vi "管理员面板.vi"() -> ()   [LabVIEW 2019]
panel:
  out "错误输出 3":errorcluster caption="错误输出"
  out "Row":i32
  out "Column":i32
  out "error out 7":errorcluster
  out "当前选择的用户为":string
  in  "重置密码":bool
  in  "删除用户":bool
  out "成员名单":string[][](table)
  out "成员名单1":string[][](array[string])
  out "error out 4":errorcluster
  in  "返回":bool
  # "欢迎来到管理员面板"
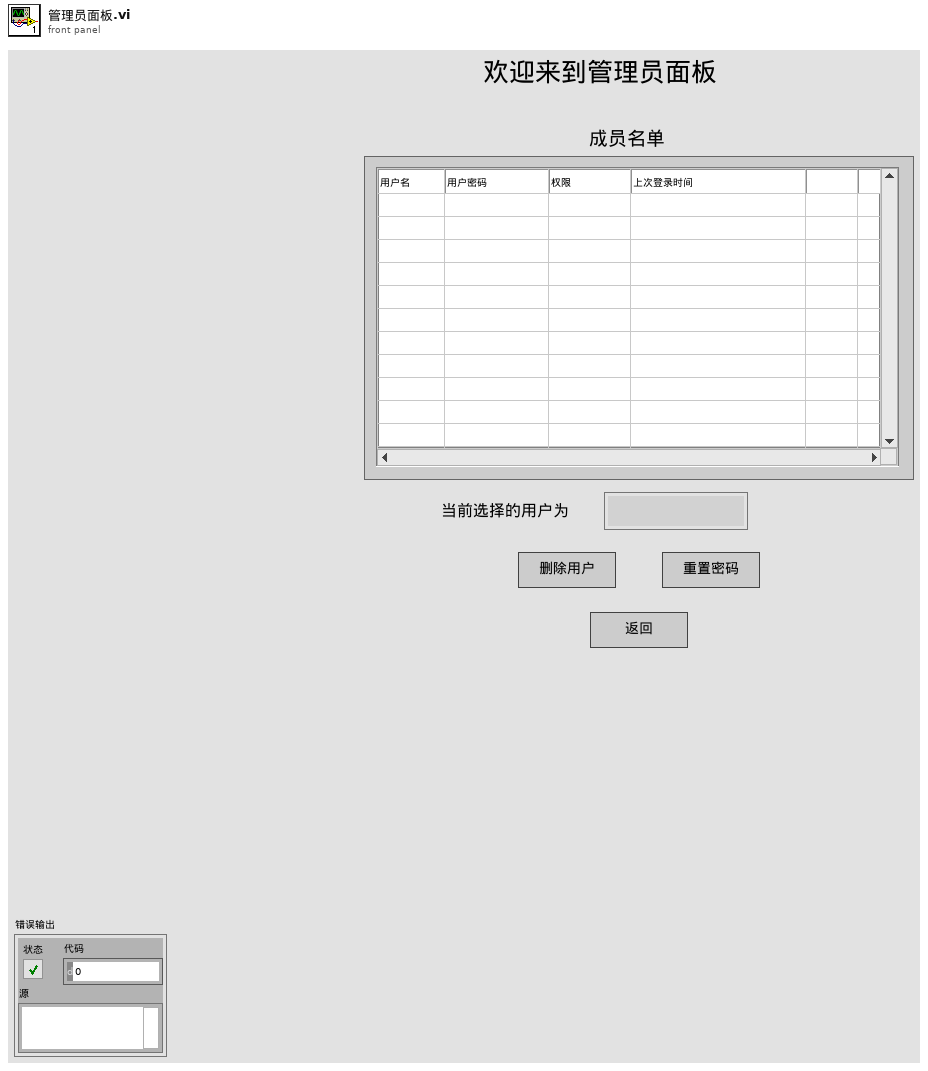
[diagram p1: front panel]
types:
  T1 = cluster{"Read Access":enum8{"Allowed", "Required", "None"}, "Write Access":enum8{"Allowed", "Required", "None"}}
  T2 = typedef "LVPoint32TypeDef.ctl" = cluster{"Horizontal":i32, "Vertical":i32}
  T3 = typedef "LVRowAndColumnTypeDef.ctl" = cluster{"Row":i32, "Column":i32}
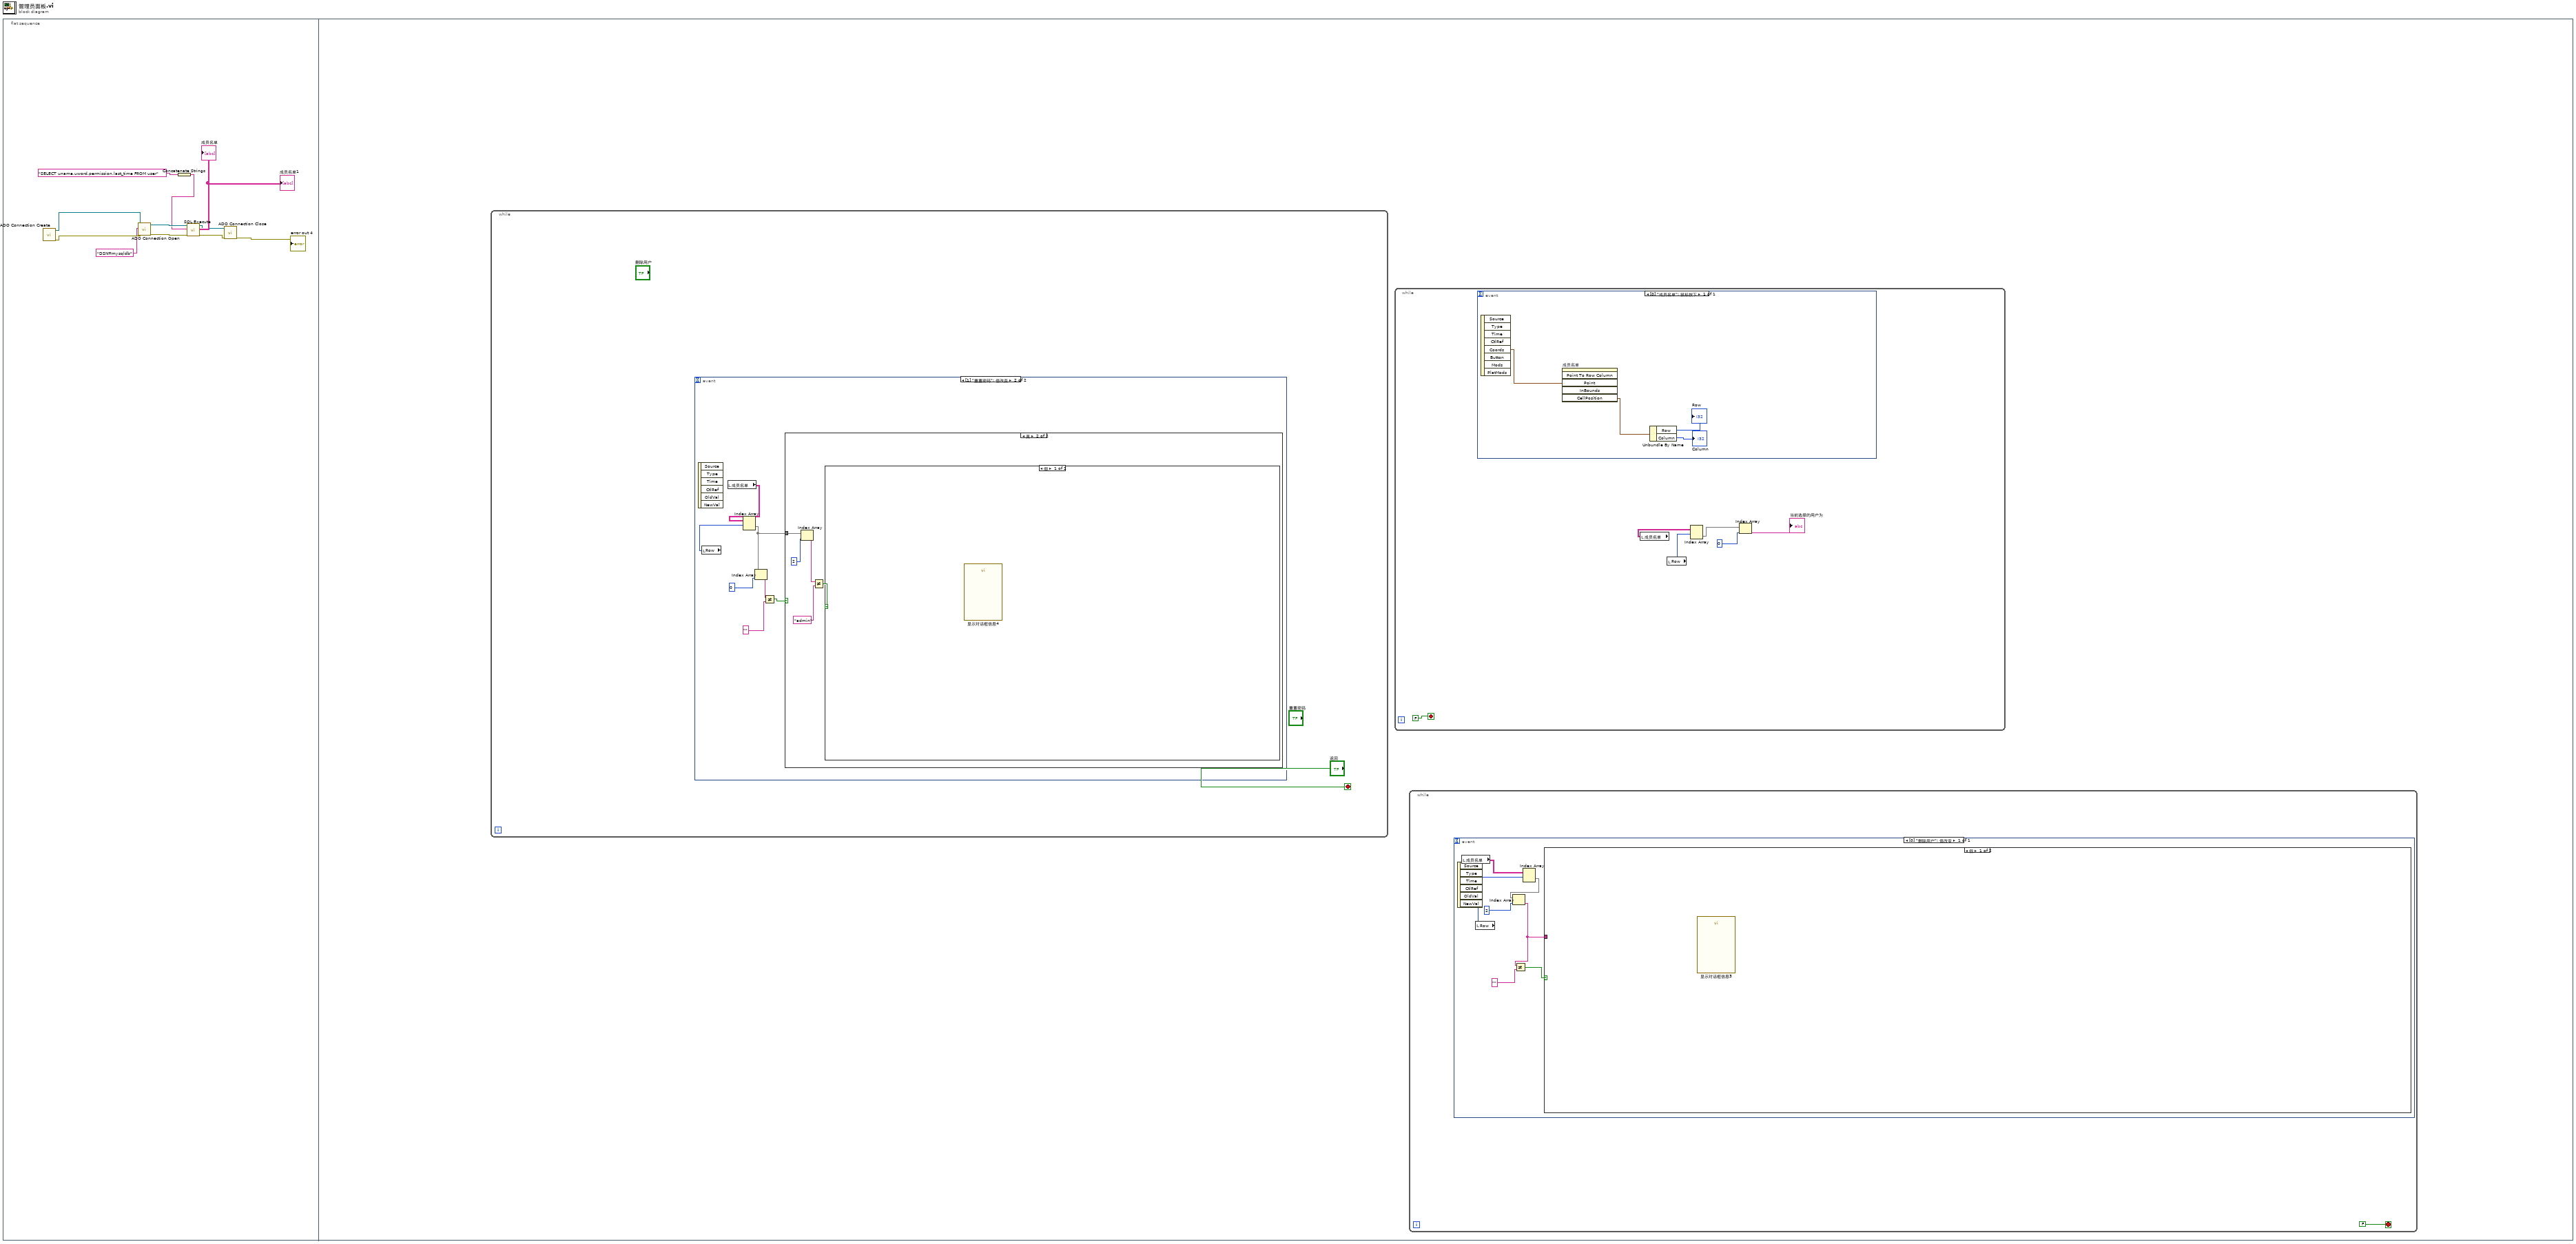
[diagram p0: block diagram]
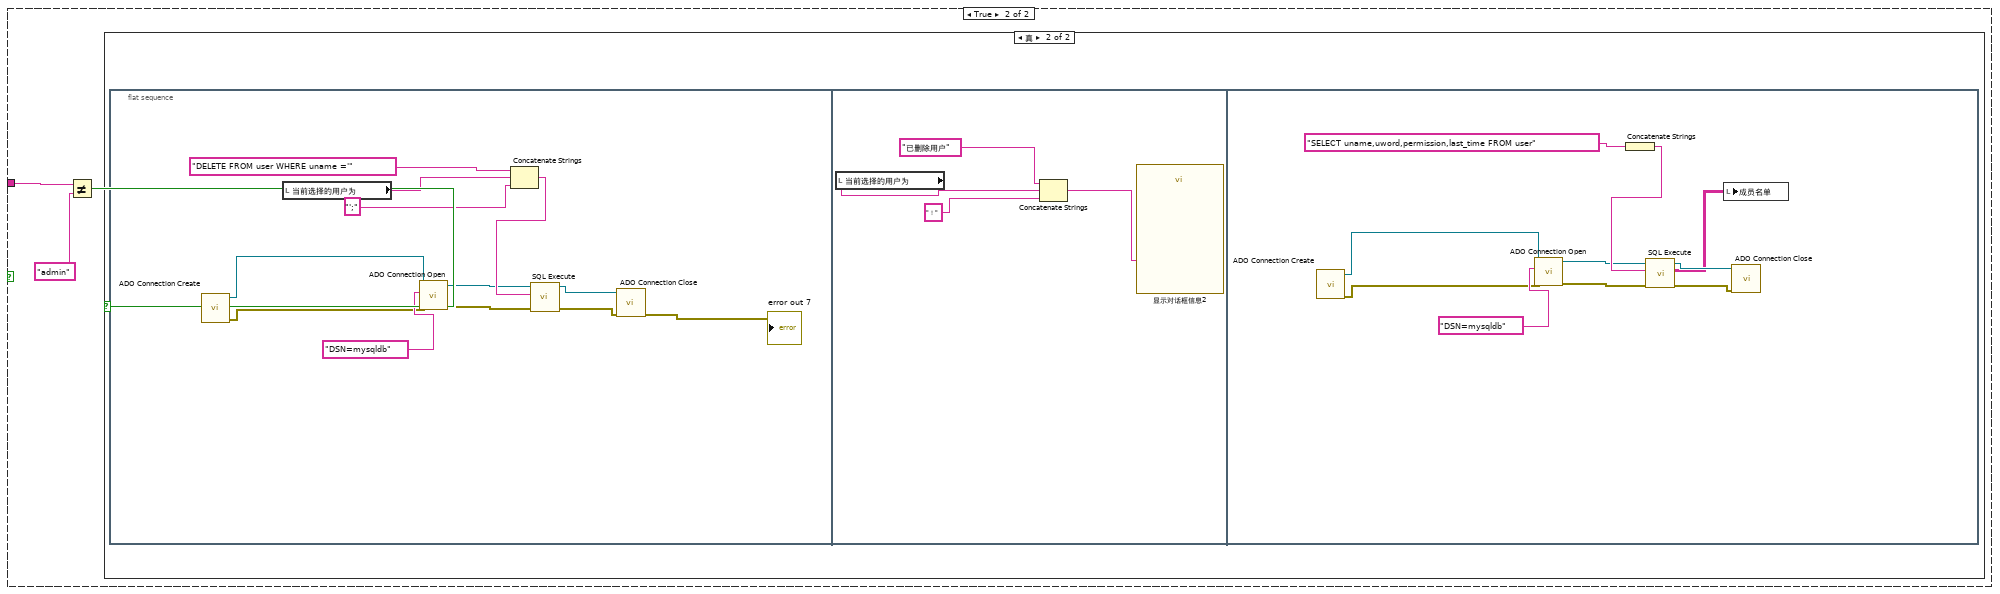
[diagram p2: hidden frame]
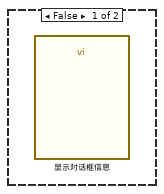
[diagram p3: hidden frame]
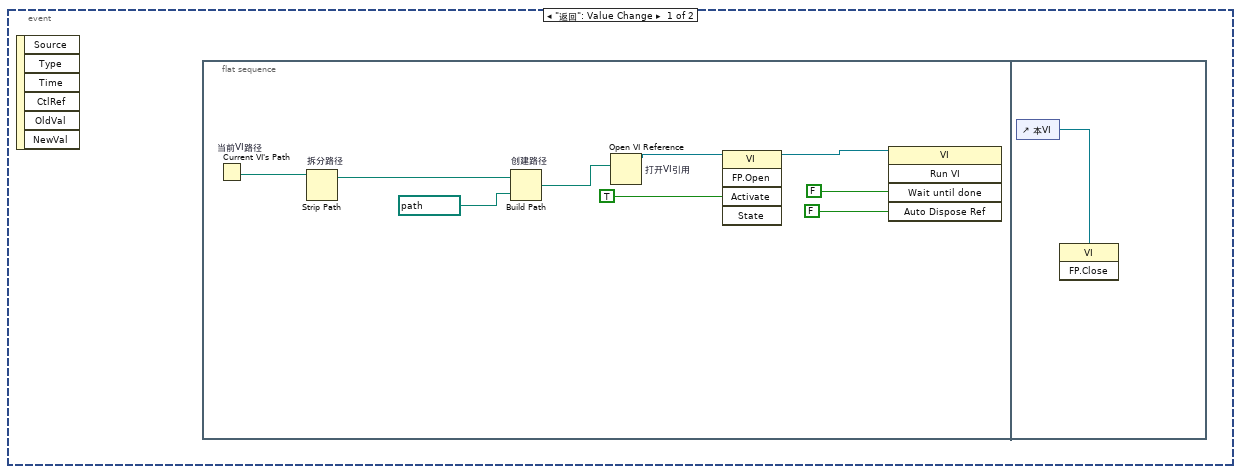
[diagram p4: hidden frame]
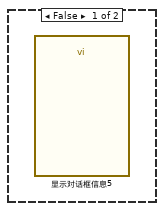
[diagram p5: hidden frame]
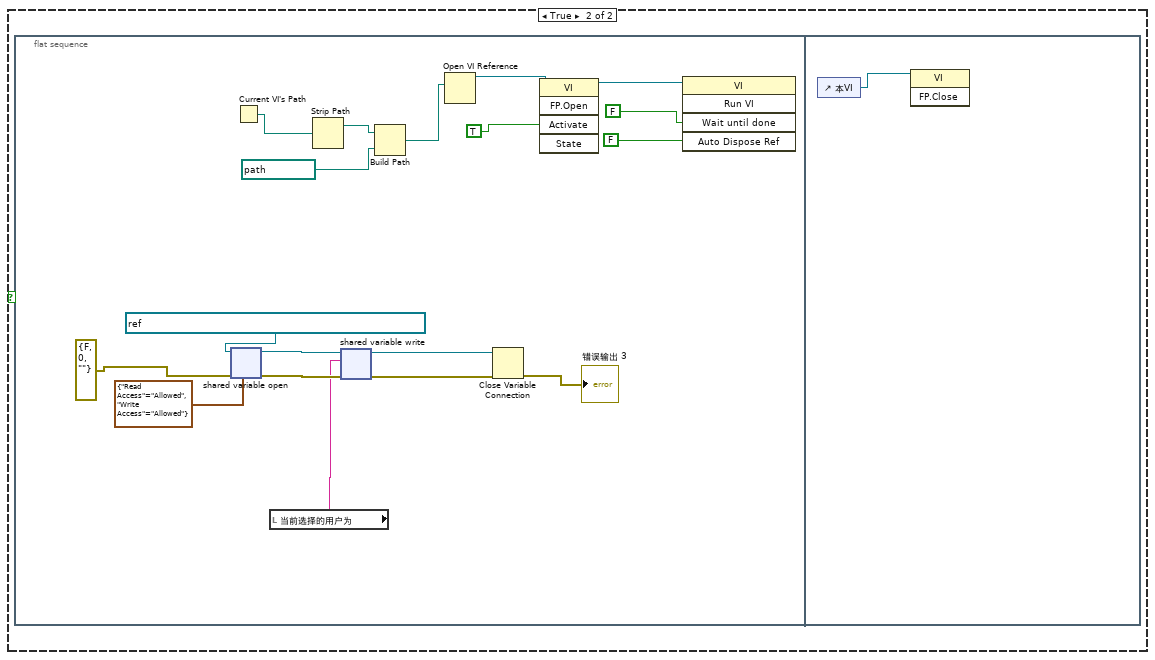
[diagram p6: hidden frame]
diagram:
  n1 = flat-sequence {
    frame #0 {
      n2 = call <userlib>:"ADO Connection Create.vi"() -> ("error out"=w9:errorcluster, "ADODB._Connection Out"=w10:refnum<k7>)  [unwired: 10 in]
      n3 = call <userlib>:"ADO Connection Open.vi"("error in (no error)"=w9, "ConnectionString"="DSN=mysqldb", "ADODB._Connection In"=w10) -> ("error out"=w8:errorcluster, "ADODB._Connection Out"=w4:refnum<k7>)  [unwired: 7 in]
      n4 = Concatenate Strings("SELECT uname,uword,permission,last_time FROM user") -> (w3:string)
      n5 = call <userlib>:"SQL Execute.vi"("error in (no error)"=w8, "Command Text"=w3, "ADODB._Connection In"=w4) -> ("error out"=w6:errorcluster, "Data"=→"成员名单1" →"成员名单":string[][], "ADODB._Connection Out"=w5:refnum<k7>)  [unwired: 5 in, 1 out]
      n6 = call <userlib>:"ADO Connection Close.vi"("error in (no error)"=w6, "ADODB._Connection In"=w5) -> ("error out"=→"error out 4":errorcluster)  [unwired: 8 in, 1 out]
    }
    frame #1 {
      n7 = while {
        stop <- "返回" stop-if-true
        n8 = event shown="[1] \"重置密码\": 值改变" {
          selector: _ -> [_ _]
          dyn-events: _ -> [_ _]
          timeout: _ -> [_ _]
          event "返回": Value Change {
            n9 = event-data() -> ()  [unwired: 1 in, 6 out]
            n10 = flat-sequence {
              frame #0 {
                n11 = Current VI's Path "当前VI路径"() -> (path=w61:path)
                n12 = Strip Path "拆分路径"(path=w61) -> (stripped path=w60:path)  [unwired: 1 out]
                n13 = Build Path "创建路径"(base path=w60, name or relative path=path "登陆后.vi") -> (appended path=w63:path)
                n14 = Open VI Reference "打开VI引用"(vi path=w63) -> (vi reference=w62:refnum<vi>)  [unwired: 5 in, 1 out]
                n15 = invoke class="VI" method="FP.Open"(reference=w62, "Activate"=TRUE) -> (reference out=w66:refnum<vi>)  [unwired: 3 in, 4 out]
                n16 = invoke class="VI" method="Run VI"(reference=w66, "Wait until done"=FALSE, "Auto Dispose Ref"=FALSE) -> ()  [unwired: 2 in, 5 out]
              }
              frame #1 {
                n17 = control-ref of="本VI"() -> (w69:refnum<vi>)
                n18 = invoke class="VI" method="FP.Close"(reference=w69) -> ()  [unwired: 2 in, 3 out]
              }
            }
          }
          event "重置密码": Value Change {
            n19 = event-data() -> ()  [unwired: 1 in, 6 out]
            n20 = local read "Row"() -> (w75:i32)
            n21 = local read "成员名单"() -> (w76:string[][])
            n22 = Index Array(array=w76, index (row)=w75) -> (element=w70:string[])  [unwired: 1 in]
            n23 = Index Array(array=w70, index=0) -> (element=w72:string)
            n24 = Not Equal?(x=w72, y="") -> (x != y?=w71:bool)
            n25 = case shown="真" w71 {
              tunnel: w70 -> [_ w77]
              frame False {
                n26 = call "显示对话框信息5"() -> ()  [unwired: 10 in, 2 out]
              }
              frame True {
                n27 = Index Array(array=w77, index=2) -> (element=w78:string)
                n28 = Not Equal?(x=w78, y="admin") -> (x != y?=w80:bool)
                n29 = case shown="假" w80 {
                  frame False {
                    n30 = call "显示对话框信息4"() -> ()  [unwired: 10 in, 2 out]
                  }
                  frame True {
                    n31 = flat-sequence {
                      frame #0 {
                        n32 = shared-variable-open(refnum<k21> "ni.var.psp://localhost/登录/管理员选择用户" ("共享变量引用句柄输入"), errorcluster {"status"=FALSE, "code"=0, "source"=""} ("错误输入（无错误）"), T1 {"Read Access"=enum."Allowed", "Write Access"=enum."Allowed"} ("权限")) -> (w90:refnum<k21>, w87:errorcluster)
                        n33 = Current VI's Path() -> (path=w94:path)
                        n34 = local read "当前选择的用户为"() -> (w82:string)
                        n35 = Strip Path(path=w94) -> (stripped path=w93:path)  [unwired: 1 out]
                        n36 = shared-variable-write(w90, w87, w82) -> (w89:refnum<k21>, w88:errorcluster)
                        n37 = Build Path(base path=w93, name or relative path=path "密码重置.vi") -> (appended path=w91:path)
                        n38 = Open VI Reference(vi path=w91) -> (vi reference=w95:refnum<vi>)  [unwired: 5 in, 1 out]
                        n39 = Close Variable Connection(8:w88, 11:w89) -> (0:→"错误输出 3":errorcluster)
                        n40 = invoke class="VI" method="FP.Open"(reference=w95, "Activate"=TRUE) -> (reference out=w96:refnum<vi>)  [unwired: 3 in, 4 out]
                        n41 = invoke class="VI" method="Run VI"(reference=w96, "Wait until done"=FALSE, "Auto Dispose Ref"=FALSE) -> ()  [unwired: 2 in, 5 out]
                      }
                      frame #1 {
                        n42 = control-ref of="本VI"() -> (w100:refnum<vi>)
                        n43 = invoke class="VI" method="FP.Close"(reference=w100) -> ()  [unwired: 2 in, 3 out]
                      }
                    }
                  }
                }
              }
            }
          }
        }
      }
      n44 = while {
        stop <- FALSE stop-if-true
        n45 = event shown="[0] \"成员名单\": 鼠标按下" {
          selector: _ -> [_]
          dyn-events: _ -> [_]
          timeout: _ -> [_]
          event "成员名单": Mouse Down {
            n46 = event-data() -> ("Coords"=w58:T2)  [unwired: 1 in, 7 out]
            n47 = invoke on="成员名单" class="Tbl (严格)" method="Point To Row Column"("Point"=w58) -> ("CellPosition"=w57:T3)  [unwired: 5 in, 5 out]
            n48 = Unbundle By Name(w57) -> ("Row"=→"Row":i32, "Column"=→"Column":i32)
          }
        }
        n49 = local read "成员名单"() -> (w54:string[][])
        n50 = local read "Row"() -> (w50:i32)
        n51 = Index Array(array=w54, index (row)=w50) -> (element=w51:string[])  [unwired: 1 in]
        n52 = Index Array(array=w51, index=0) -> (element=→"当前选择的用户为":string)
      }
      n53 = while {
        stop <- FALSE stop-if-true
        n54 = event shown="[0] \"删除用户\": 值改变" {
          selector: _ -> [_]
          dyn-events: _ -> [_]
          timeout: _ -> [_]
          event "删除用户": Value Change {
            n55 = event-data() -> ()  [unwired: 1 in, 6 out]
            n56 = local read "成员名单"() -> (w18:string[][])
            n57 = local read "Row"() -> (w17:i32)
            n58 = Index Array(array=w18, index (row)=w17) -> (element=w16:string[])  [unwired: 1 in]
            n59 = Index Array(array=w16, index=2) -> (element=w13:string)
            n60 = Not Equal?(x=w13, y="") -> (x != y?=w14:bool)
            n61 = case shown="假" w14 {
              tunnel: w13 -> [_ w22]
              frame False {
                n62 = call "显示对话框信息3"() -> ()  [unwired: 10 in, 2 out]
              }
              frame True {
                n63 = Not Equal?(x=w22, y="admin") -> (x != y?=w21:bool)
                n64 = case shown="真" w21 {
                  frame False {
                    n65 = call "显示对话框信息"() -> ()  [unwired: 10 in, 2 out]
                  }
                  frame True {
                    n66 = flat-sequence {
                      frame #0 {
                        n67 = call <userlib>:"ADO Connection Create.vi"() -> ("error out"=w26:errorcluster, "ADODB._Connection Out"=w25:refnum<k7>)  [unwired: 10 in]
                        n68 = local read "当前选择的用户为"() -> (w23:string)
                        n69 = call <userlib>:"ADO Connection Open.vi"("error in (no error)"=w26, "ConnectionString"="DSN=mysqldb", "ADODB._Connection In"=w25) -> ("error out"=w29:errorcluster, "ADODB._Connection Out"=w33:refnum<k7>)  [unwired: 7 in]
                        n70 = Concatenate Strings("DELETE FROM user WHERE uname ='", w23, "';") -> (w34:string)
                        n71 = call <userlib>:"SQL Execute.vi"("error in (no error)"=w29, "Command Text"=w34, "ADODB._Connection In"=w33) -> ("error out"=w31:errorcluster, "ADODB._Connection Out"=w32:refnum<k7>)  [unwired: 5 in, 2 out]
                        n72 = call <userlib>:"ADO Connection Close.vi"("error in (no error)"=w31, "ADODB._Connection In"=w32) -> ("error out"=→"error out 7":errorcluster)  [unwired: 8 in, 1 out]
                      }
                      frame #1 {
                        n73 = local read "当前选择的用户为"() -> (w35:string)
                        n74 = Concatenate Strings("已删除用户", w35, "！") -> (w36:string)
                        n75 = call "显示对话框信息2"("Message"=w36) -> ()  [unwired: 9 in, 2 out]
                      }
                      frame #2 {
                        n76 = call <userlib>:"ADO Connection Create.vi"() -> ("error out"=w42:errorcluster, "ADODB._Connection Out"=w41:refnum<k7>)  [unwired: 10 in]
                        n77 = call <userlib>:"ADO Connection Open.vi"("error in (no error)"=w42, "ConnectionString"="DSN=mysqldb", "ADODB._Connection In"=w41) -> ("error out"=w44:errorcluster, "ADODB._Connection Out"=w47:refnum<k7>)  [unwired: 7 in]
                        n78 = Concatenate Strings("SELECT uname,uword,permission,last_time FROM user") -> (w48:string)
                        n79 = call <userlib>:"SQL Execute.vi"("error in (no error)"=w44, "Command Text"=w48, "ADODB._Connection In"=w47) -> ("error out"=w45:errorcluster, "Data"=w39:string[][], "ADODB._Connection Out"=w46:refnum<k7>)  [unwired: 5 in, 1 out]
                        n80 = local write "成员名单"(w39) -> ()
                        n81 = call <userlib>:"ADO Connection Close.vi"("error in (no error)"=w45, "ADODB._Connection In"=w46) -> ()  [unwired: 8 in, 2 out]
                      }
                    }
                  }
                }
              }
            }
          }
        }
      }
    }
  }
